vi "Clean Build Artifacts.vi"(0 "NI Build Specification in":refnum<class "Installer_LV.lvclass">, 11 "error in (no error)":errorcluster) -> (4 "NI Build Specification out":refnum<class "Installer_LV.lvclass">, 15 "error out":errorcluster)   [LabVIEW 2017, in "CL_G3_VIComponentBuilder.lvlib" / "Installer_LV.lvclass"]
doc: "Deletes the installer at the location specified by the Installer Destination of the build specification."
uses:
  Installer_LV.lvclass
  C:/builds/Component BuilderBT/SrcDist/Exports/Exports/Export.lvclass
  Exports/Export.lvclass/Export.ctl
  Exports/Accessors/Read Exported Build Specification Path.vi
  <vilib>/xml/Load XML File.vi
  <vilib>/xml/Close Reference(Node).vi
  NI Build Specification_LV/NI Build Specification_LV.lvclass
  <vilib>/xml/NI_XML.lvlib
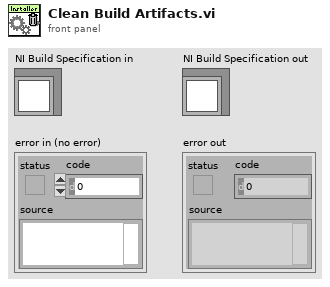
[diagram p1: front panel]
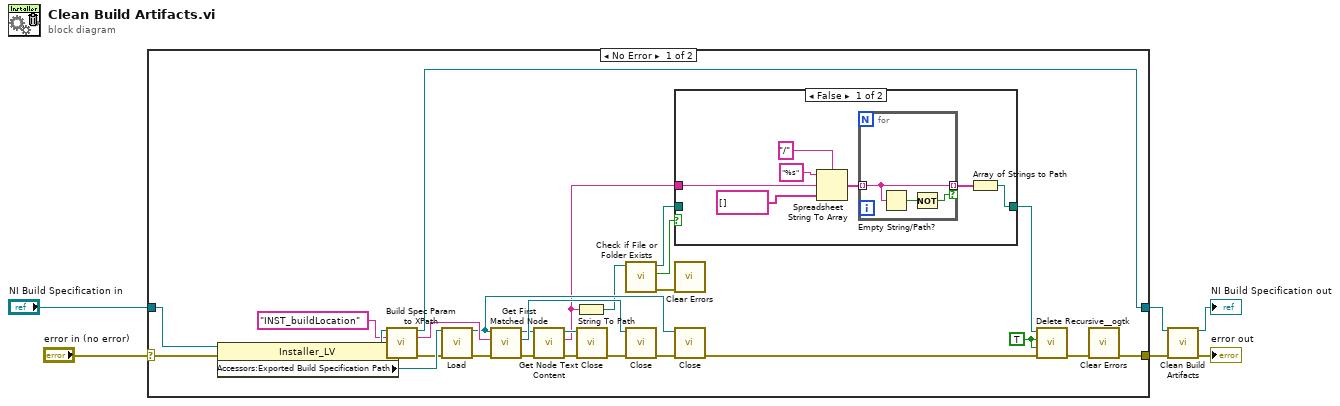
[diagram p0: block diagram]
diagram:
  n1 = case shown="No Error" "error in (no error)" {
    selector: "error in (no error)" -> [w27 w46]
    tunnel: "NI Build Specification in" -> [w28 w47]
    tunnel: [w10 w47] -> w2
    tunnel: [w7 w46] -> w4
    frame No Error {
      w12 = TRUE ("Recursive? (FALSE)")
      n2 = property class="Installer_LV"(reference=w28, error in=w27) -> (reference out=w32:refnum<class "Installer_LV.lvclass">, error out=w30:errorcluster, "Accessors:Exported Build Specification Path"=w33:path)
      n3 = call-dynamic "Build Spec Param to XPath.vi"("NI Build Specification"=w32, "Build Spec Parameter Name"="INST_buildLocation", "error in (no error)"=w30) -> ("NI Build Specification"=w10:refnum<class "Installer_LV.lvclass">, "XPath to the specific build Spec Property"=w31:string, "error out"=w29:errorcluster)  [unwired: 10 in]
      n4 = call-poly <vilib>:"Load.vi"("path to XML document"=w33, "error in (no error)"=w29) -> ("DOM document out"=w25:refnum<k20>, "error out"=w34:errorcluster)  [unwired: 11 in, 1 out]
      n5 = call <vilib>:"Get First Matched Node.vi"("error in (no error)"=w34, "XPath expression"=w31, "node in"=w25) -> ("error out"=w22:errorcluster, "node result"=w24:refnum<k20>, "node out"=w23:refnum<k20>)  [unwired: 6 in]
      n6 = call <vilib>:"Get Node Text Content.vi"("error in (no error)"=w22, "node in"=w23) -> ("error out"=w21:errorcluster, "node text"=w14:string, "node out"=w20:refnum<k20>)  [unwired: 7 in]
      n7 = String To Path(string=w14) -> (path=w18:path)
      n8 = call-poly <vilib>:"Close.vi"("error in (no error)"=w21, "node"=w20) -> ("error out"=w19:errorcluster)  [unwired: 7 out]
      n9 = call <vilib>:"Check if File or Folder Exists.vi"("path"=w18) -> ("error out"=w15:errorcluster, "file or folder exists?"=w17:bool, "dup path"=w16:path)  [unwired: 8 in]
      n10 = call-poly <vilib>:"Close.vi"("error in (no error)"=w19, "node"=w24) -> ("error out"=w26:errorcluster)  [unwired: 7 out]
      n11 = case shown="False" w17 {
        tunnel: [w36 w45] -> w13
        tunnel: w14 -> [w35 _]
        tunnel: w16 -> [_ w45]
        frame False {
          n12 = Spreadsheet String To Array(delimiter (Tab)="/", format string="%s", spreadsheet string=w35, array type (2D Dbl)=string[] []) -> (array=w40:string[])
          n13 = for {
            tunnel: w40 -> [w43] mode=indexing
            tunnel: [w43] -> w41 mode=indexing if=w42
            n14 = Empty String/Path?(string/path=w43) -> (empty?=w44:bool)
            n15 = Not(x=w44) -> (.not. x?=w42:bool)
          }
          n16 = Array of Strings to Path(0:w41) -> (2:w36:path)  [unwired: 1 in]
        }
        frame True {
        }
      }
      n17 = call <vilib>:"Clear Errors.vi"("error in (no error)"=w15) -> ()  [unwired: 5 in, 2 out]
      n18 = call-poly <vilib>:"Close.vi"("error in (no error)"=w26, "node"=w25) -> ("error out"=w11:errorcluster)  [unwired: 7 in]
      n19 = call <userlib>:"Delete Recursive__ogtk.vi"("error in (no error)"=w11, "Ignore Read-Only? (FALSE)"=w12, "Recursive? (FALSE)"=w12, "Path"=w13) -> ("error out"=w9:errorcluster)  [unwired: 6 in, 1 out]
      n20 = call <vilib>:"Clear Errors.vi"("error in (no error)"=w9) -> ("error out"=w7:errorcluster)  [unwired: 5 in, 1 out]
    }
    frame Error {
    }
  }
  n21 = call-parent "Clean Build Artifacts.vi"("NI Build Specification in"=w2, "error in (no error)"=w4) -> ("NI Build Specification out"=→"NI Build Specification out":refnum<class "Installer_LV.lvclass">, "error out"=→"error out":errorcluster)  [unwired: 12 in]
